vi "Write to String Log.vi"(10 "String to Log":string, 11 "Text File Sink in":refnum<class "Text File Sink.lvclass">) -> (0 "error out":errorcluster, 3 "Text File Sink out":refnum<class "Text File Sink.lvclass">)   [LabVIEW 2017, in "Text File Sink.lvclass"]
uses:
  Text File Sink.lvclass
  Text File Sink.lvclass/Text File Sink.ctl
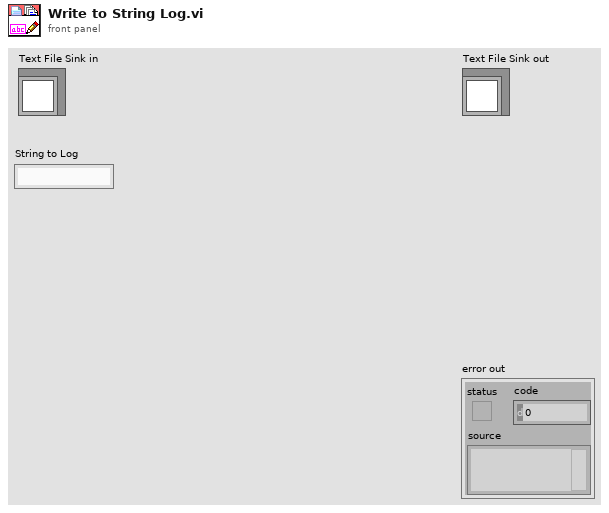
[diagram p1: front panel]
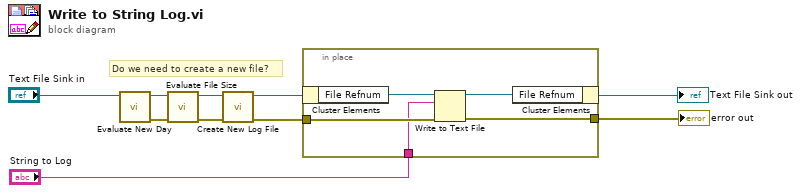
[diagram p0: block diagram]
diagram:
  # "Do we need to create a new file?"
  n1 = call "Evaluate New Day.vi"("Text File Sink in"="Text File Sink in") -> ("error out"=w8:errorcluster, "Text File Sink out"=w10:refnum<class "Text File Sink.lvclass">)  [unwired: 9 in]
  n2 = call "Evaluate File Size.vi"("error in (no error)"=w8, "Text File Sink in"=w10) -> ("error out"=w7:errorcluster, "Text File Sink out"=w9:refnum<class "Text File Sink.lvclass">)  [unwired: 8 in]
  n3 = call "Create New Log File.vi"("error in (no error)"=w7, "Text File Sink in"=w9) -> ("error out"=w3:errorcluster, "Text File Sink out"=w5:refnum<class "Text File Sink.lvclass">)  [unwired: 8 in]
  n4 = in-place {
    in-place-border: w3 -> [w13]
    in-place-border: [w12] -> w2
    in-place-border: "String to Log" -> [w11]
    n5 = in-place-cluster #1(w5) -> ("File Refnum"=w15:refnum<file>)
    n6 = Write to Text File(file (use dialog)=w15, text=w11, error in=w13) -> (refnum out=w14:refnum<file>, error out=w12:errorcluster)  [unwired: 2 out]
    n7 = in-place-cluster #1("File Refnum"=w14) -> (→"Text File Sink out":refnum<class "Text File Sink.lvclass">)
  }
  "error out" <- w2
